vi "Rename Dynamic Dispatch Member.vi"(8 "error in (no error)":errorcluster, 10 "new name":string, 11 "vi in":refnum<vi>) -> (0 "error out":errorcluster, 1 "refactor result":T1, 2 "additional mapping info":T2)   [LabVIEW 2020, in "MeasurementService Editor.lvlib"]
uses:
  MeasurementService Editor.lvlib
  Rename Refactor Mapping Info.ctl
  Refactor Dynamic Dispatch Member Result.ctl
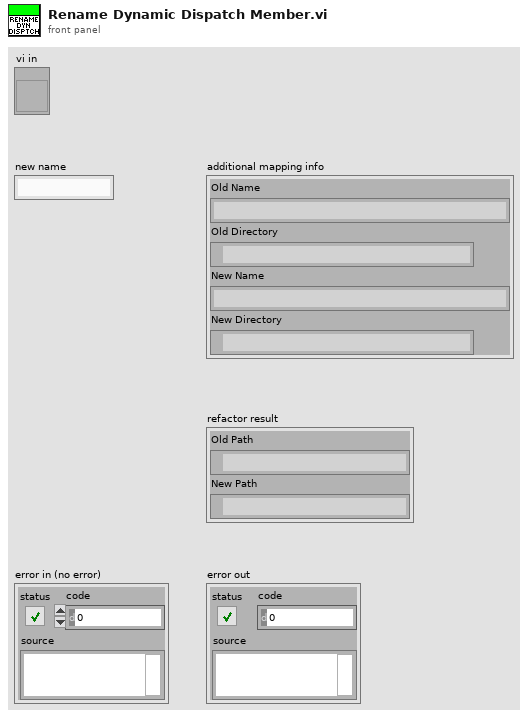
[diagram p1: front panel]
types:
  T1 = typedef "MeasurementService Editor.lvlib/Refactor Dynamic Dispatch Member Result.ctl" = cluster{"Old Path":path, "New Path":path}
  T2 = typedef "MeasurementService Editor.lvlib/Rename Refactor Mapping Info.ctl" = cluster{"Old Name":string, "Old Directory":path, "New Name":string, "New Directory":path}
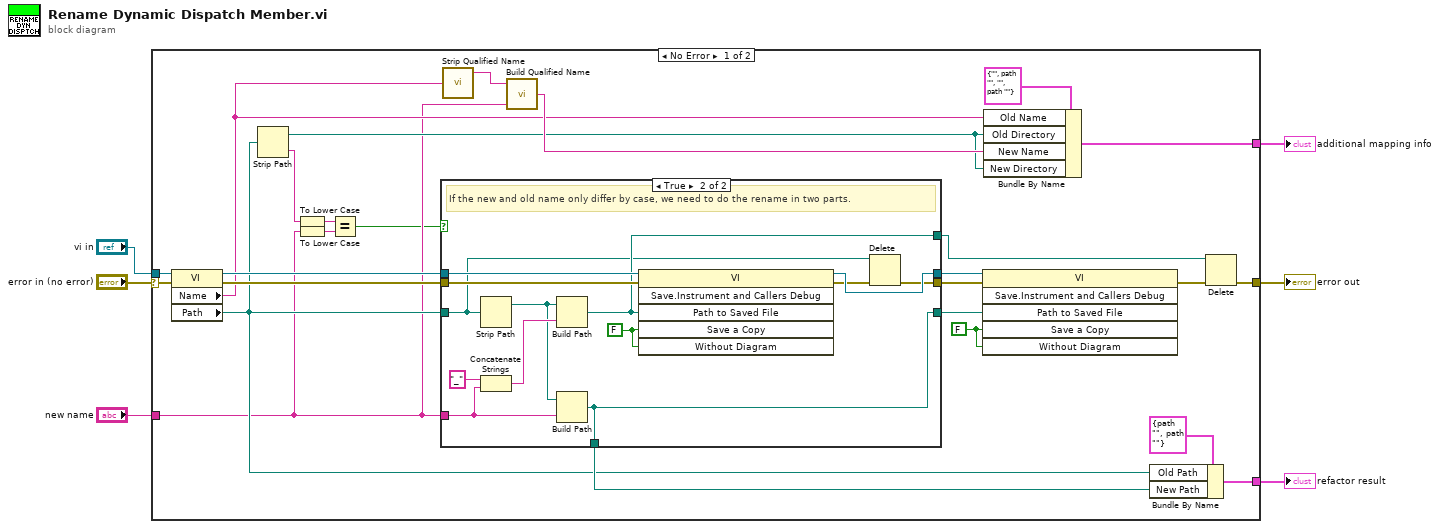
[diagram p0: block diagram]
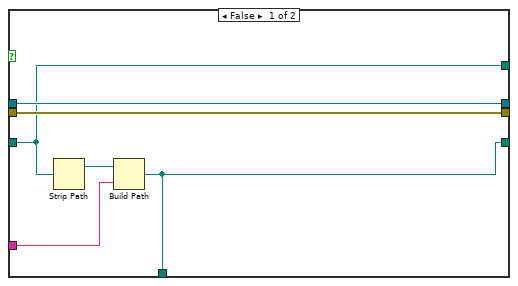
[diagram p2: hidden frame]
diagram:
  n1 = case shown="No Error" "error in (no error)" {
    selector: "error in (no error)" -> [w17 w52]
    tunnel: "vi in" -> [w15 _]
    tunnel: "new name" -> [w9 _]
    tunnel: [w30 w52] -> w4
    tunnel: [w28 _] -> w3
    tunnel: [w18 _] -> w6
    frame No Error {
      w32 = FALSE ("Save a Copy")
      n2 = property class="VI"(reference=w15, error in=w17) -> (reference out=w14:refnum<vi>, error out=w16:errorcluster, "Name"=w13:string, "Path"=w12:path)
      n3 = Strip Path(path=w12) -> (stripped path=w19:path, name=w10:string)
      n4 = To Lower Case(string=w10) -> (all lower case string=w7:string)
      n5 = To Lower Case(string=w9) -> (all lower case string=w11:string)
      n6 = Equal?(x=w7, y=w11) -> (x = y?=w8:bool)
      n7 = case shown="True" w8 {
        tunnel: w14 -> [w36 w50]
        tunnel: w16 -> [w35 w49]
        tunnel: [w35 w40] -> w27
        tunnel: [w36 w48] -> w26
        tunnel: [w34 w42] -> w25
        tunnel: w9 -> [w37 w43]
        tunnel: w12 -> [w33 w39]
        tunnel: [w34 w42] -> w24
        tunnel: [w33 w45] -> w23
        frame False {
          n8 = Strip Path(path=w33) -> (stripped path=w38:path)  [unwired: 1 out]
          n9 = Build Path(base path=w38, name or relative path=w37) -> (appended path=w34:path)
        }
        frame True {
          w51 = FALSE ("Save a Copy")
          # "If the new and old name only differ by case, we need to do the rename in two parts."
          n10 = Strip Path(path=w39) -> (stripped path=w44:path)  [unwired: 1 out]
          n11 = Concatenate Strings("_" ("string"), w43) -> (w46:string)
          n12 = Build Path(base path=w44, name or relative path=w46) -> (appended path=w45:path)
          n13 = Build Path(base path=w44, name or relative path=w43) -> (appended path=w42:path)
          n14 = invoke class="VI" method="Save.Instrument and Callers Debug"(reference=w50, error in=w49, "Path to Saved File"=w45, "Save a Copy"=w51, "Without Diagram"=w51) -> (reference out=w48:refnum<vi>, error out=w41:errorcluster)  [unwired: 1 in, 4 out]
          n15 = Delete(path (use dialog)=w39, error in=w41) -> (error out=w40:errorcluster)  [unwired: 3 in, 2 out]
        }
      }
      n16 = call "Strip Qualified Name.vi"("name"=w13) -> ("stripped name"=w21:string)  [unwired: 5 in, 1 out]
      n17 = call "Build Qualified Name.vi"("name"=w9, "base name"=w21) -> ("appended name"=w20:string)  [unwired: 3 in]
      n18 = invoke class="VI" method="Save.Instrument and Callers Debug"(reference=w26, error in=w27, "Path to Saved File"=w25, "Save a Copy"=w32, "Without Diagram"=w32) -> (error out=w31:errorcluster)  [unwired: 1 in, 5 out]
      n19 = Bundle By Name(cluster=T2 {"Old Name"="", "Old Directory"=path "", "New Name"="", "New Directory"=path ""} ("Rename Mapping Info"), "Old Name"=w13, "Old Directory"=w19, "New Name"=w20, "New Directory"=w19) -> (w18:T2)
      n20 = Bundle By Name(cluster=T1 {"Old Path"=path "", "New Path"=path ""} ("Refactor Dynamic Dispatch Member Result"), "Old Path"=w12, "New Path"=w24) -> (w28:T1)
      n21 = Delete(path (use dialog)=w23, error in=w31) -> (error out=w30:errorcluster)  [unwired: 3 in, 2 out]
    }
    frame Error {
    }
  }
  "additional mapping info" <- w6
  "error out" <- w4
  "refactor result" <- w3
